vi "myRIO_BRig_RT_dataExp_init.vi"() -> (3 "output_dataExp":u16[](array[numeric]))   [LabVIEW 2014]
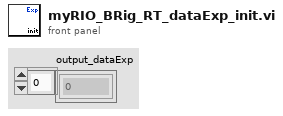
[diagram p1: front panel]
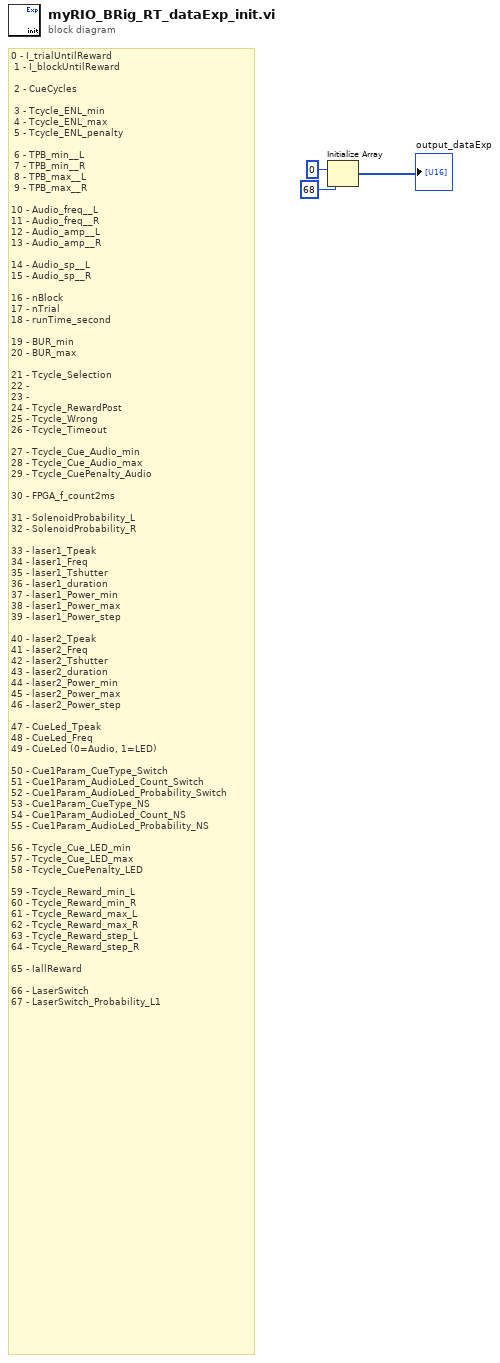
[diagram p0: block diagram]
diagram:
  # "0 - I_trialUntilReward\n 1 - I_blockUntilReward\n\n 2 - CueCycles\n\n 3 - Tcycle_ENL_min\n 4 - Tcycle_ENL_max\n 5 - Tcycle_ENL_penalty\n\n 6 - TPB_min__L\n 7 - TPB_min__R\n 8 - TPB_max__L\n 9 - TPB_max__R\n\n10 - Audio_freq__L\n11 - Audio_freq__R\n12 - Audio_amp__L\n13 - Audio_amp__R\n\n14 - Audio_sp__L\n15 - Audio_sp__R\n\n16 - nBlock\n17 - nTrial\n18 - runTime_second\n\n19 - BUR_min\n20 - BUR_max\n\n21 - Tcycle_Selection\n22 - \n23 - \n24 - Tcycle_RewardPost\n25 - Tcycle_Wrong\n26 - Tcycle_Timeout \n\n27 - Tcycle_Cue_Audio_min\n28 - Tcycle_Cue_Audio_max\n29 - Tcycle_CuePenalty_Audio\n\n30 - FPGA_f_count2ms\n\n31 - SolenoidProbability_L\n32 - SolenoidProbability_R\n\n33 - laser1_Tpeak\n34 - laser1_Freq\n35 - laser1_Tshutter\n36 - laser1_duration\n37 - laser1_Power_min\n38 - laser1_Power_max\n39 - laser1_Power_step\n\n40 - laser2_Tpeak\n41 - laser2_Freq\n42 - laser2_Tshutter\n43 - laser2_duration\n44 - laser2_Power_min\n45 - laser2_Power_max\n46 - laser2_Power_step\n\n47 - CueLed_Tpeak\n48 - CueLed_Freq\n49 - CueLed (0=Audio, 1=LED)\n\n50 - Cue1Param_CueType_Switch\n51 - Cue1Param_AudioLed_Count_Switch\n52 - Cue1Param_AudioLed_Probability_Switch\n53 - Cue1Param_CueType_NS\n54 - Cue1Param_AudioLed_Count_NS\n55 - Cue1Param_AudioLed_Probability_NS\n\n56 - Tcycle_Cue_LED_min\n57 - Tcycle_Cue_LED_max\n58 - Tcycle_CuePenalty_LED\n\n59 - Tcycle_Reward_min_L\n60 - Tcycle_Reward_min_R\n61 - Tcycle_Reward_max_L\n62 - Tcycle_Reward_max_R\n63 - Tcycle_Reward_step_L\n64 - Tcycle_Reward_step_R\n\n65 - IallReward\n\n66 - LaserSwitch\n67 - LaserSwitch_Probability_L1"
  n1 = Initialize Array(u16 0 ("element"), 68 ("dimension size")) -> (→"output_dataExp":u16[])
